vi "Start Trial.vi"(8 "error in (no error)":errorcluster, 10 "Trial Number":i32, 11 "NI Force Task in":refnum<class "NI Force Task.lvclass">) -> (0 "error out":errorcluster, 3 "NI Force Task out":refnum<class "NI Force Task.lvclass">)   [LabVIEW 2020, in "NI Force Task.lvlib" / "NI Force Task.lvclass"]
uses:
  NI Force Task.lvclass
  NI Force Task.lvclass/NI Force Task.ctl
  Lissajous Viewer Messages/Start Stop Trial Msg/Start Stop Trial Msg.lvclass
  Task Viewer Messages/Start Countdown Msg/Start Countdown Msg.lvclass
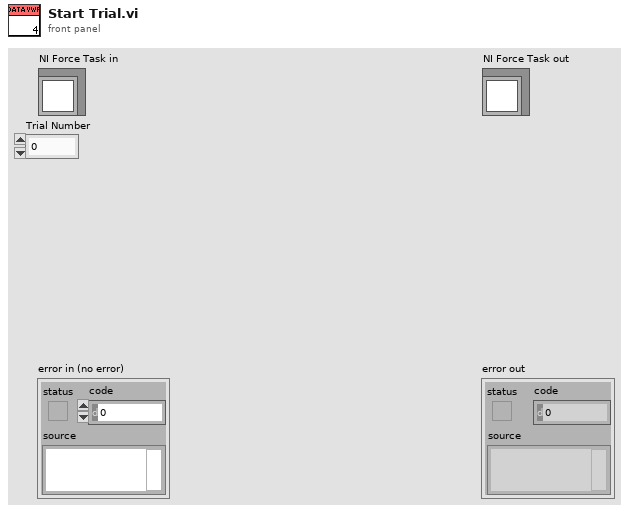
[diagram p1: front panel]
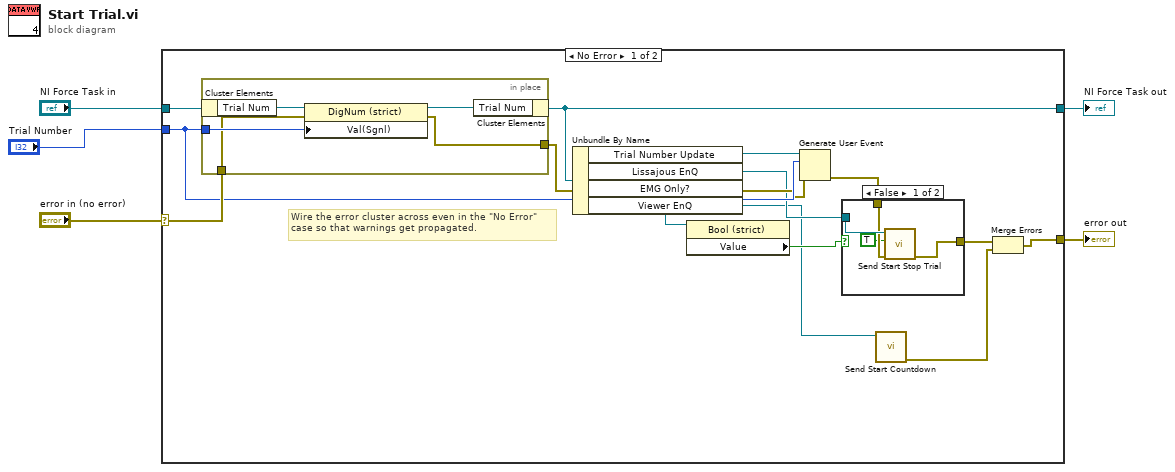
[diagram p0: block diagram]
diagram:
  n1 = case shown="No Error" "error in (no error)" {
    selector: "error in (no error)" -> [w18 w31]
    tunnel: [w7 w31] -> w4
    tunnel: [w17 w30] -> w2
    tunnel: "NI Force Task in" -> [w19 w30]
    tunnel: "Trial Number" -> [w15 _]
    frame No Error {
      # "Wire the error cluster across even in the \"No Error\"\ncase so that warnings get propagated."
      n2 = in-place {
        in-place-border: w15 -> [w27]
        in-place-border: w18 -> [w26]
        in-place-border: [w25] -> w14
        n3 = in-place-cluster #1(w19) -> ("Trial Num"=w29:refnum<vi>)
        n4 = property class="DigNum (strict)"(reference=w29, error in=w26, "Val(Sgnl)"=w27) -> (reference out=w28:refnum<vi>, error out=w25:errorcluster)
        n5 = in-place-cluster #1("Trial Num"=w28) -> (w17:refnum<class "NI Force Task.lvclass">)
      }
      n6 = Unbundle By Name(w17) -> ("Trial Number Update"=w16:refnum<user-event>, "Lissajous EnQ"=w13:refnum<class "Message Enqueuer.lvclass">, "EMG Only?"=w11:refnum<vi>, "Viewer EnQ"=w9:refnum<class "Message Enqueuer.lvclass">)
      n7 = property class="Bool (strict)"(reference=w11) -> ("Value"=w10:bool)  [unwired: 1 in, 2 out]
      n8 = Generate User Event(user event=w16, event data cluster=w15, error in=w14) -> (error out=w12:errorcluster)  [unwired: 1 in, 1 out]
      n9 = case shown="False" w10 {
        tunnel: w13 -> [w23 _]
        tunnel: [w22 w24] -> w8
        tunnel: w12 -> [w21 w24]
        frame False {
          n10 = call "Send Start Stop Trial.vi"("error in (no error)"=w21, "Acquiring true?"=TRUE, "Message Enqueuer in"=w23) -> ("error out"=w22:errorcluster)  [unwired: 7 in, 1 out]
        }
        frame True {
        }
      }
      n11 = call "Send Start Countdown.vi"("Message Enqueuer in"=w9) -> ("error out"=w6:errorcluster)  [unwired: 9 in, 1 out]
      n12 = Merge Errors(w8, w6) -> (w7:errorcluster)
    }
    frame Error {
    }
  }
  "error out" <- w4
  "NI Force Task out" <- w2
